vi "LabVIEW_Interface.vi"() -> ()   [LabVIEW 2023]
uses:
  <vilib>/Instr/_visa.llb/VISA Configure Serial Port (Instr).vi
  <vilib>/addons/control/pid/pid.llb/PID (DBL).vi
  <vilib>/addons/control/pid/NI_PID_pid.lvlib
panel:
  in  "PID/Manual control":bool
  in  "Horizontal Pointer time Arduino":i32(slide)=78 scale=20.0..100.0
  out "Microcontroller reading time":dbl(graph)=78.0
  out "Manual control":bool
  out "PID control":bool=TRUE
  in  "Third speed":i32=128 min=0 max=255 step=1
  in  "Second speed":i32=255 min=0 max=255 step=1
  in  "First speed":i32=255 min=0 max=255 step=1
  out "output manual control":i32=255
  out "Status":string="Closing connection."
  in  "PID gains":T1={"Proportional gain (Kp)"=60.0, "Integral time (Ti)"=0.2, "Derivative time (Td)"=0.0} {"Derivative time (Td)" step=0.001; "Integral time (Ti)" step=0.1; "Proportional gain (Kp)" step=0.1}
  out "output PID":i32=26
  out "Last distance value":dbl=7.16
  out "Sent target position value":dbl=7.0
  out "Vertical Graduated Bar":dbl(slide)=7.16 scale=6.0..16.0
  out "Off":bool=TRUE
  in  "Target position":dbl=7.0 min=7.0 max=16.0 step=0.1
  out "Press submit":bool=TRUE
  in  "Submit":bool
  in  "Stop":bool
  out "On":bool
  in  "VISA resource name":refnum<visa-resource-name>="COM3"
  out "Distance from the linear actuator":waveform(dbl)(graph)={"t0"=timestamp(3798521723.060967 s since 1904-01-01), "dt"=1.0, "Y"=[7.16]}
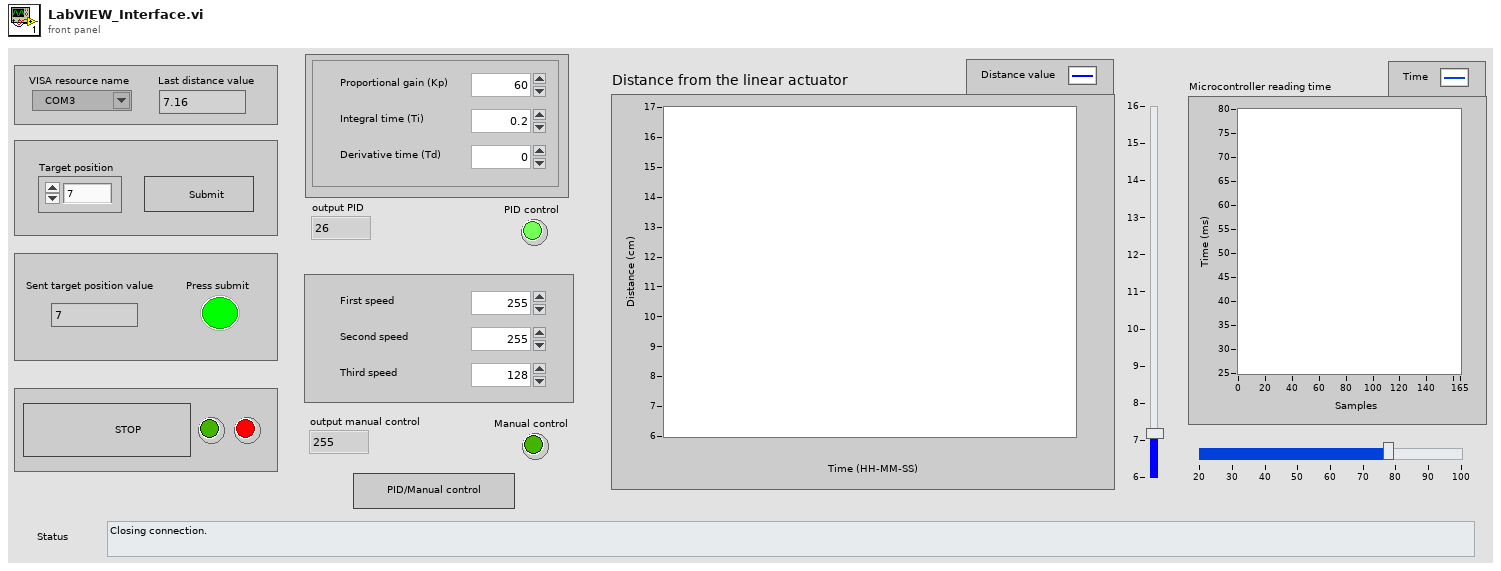
[diagram p1: front panel]
types:
  T1 = cluster{"Proportional gain (Kp)":dbl, "Integral time (Ti)":dbl, "Derivative time (Td)":dbl}
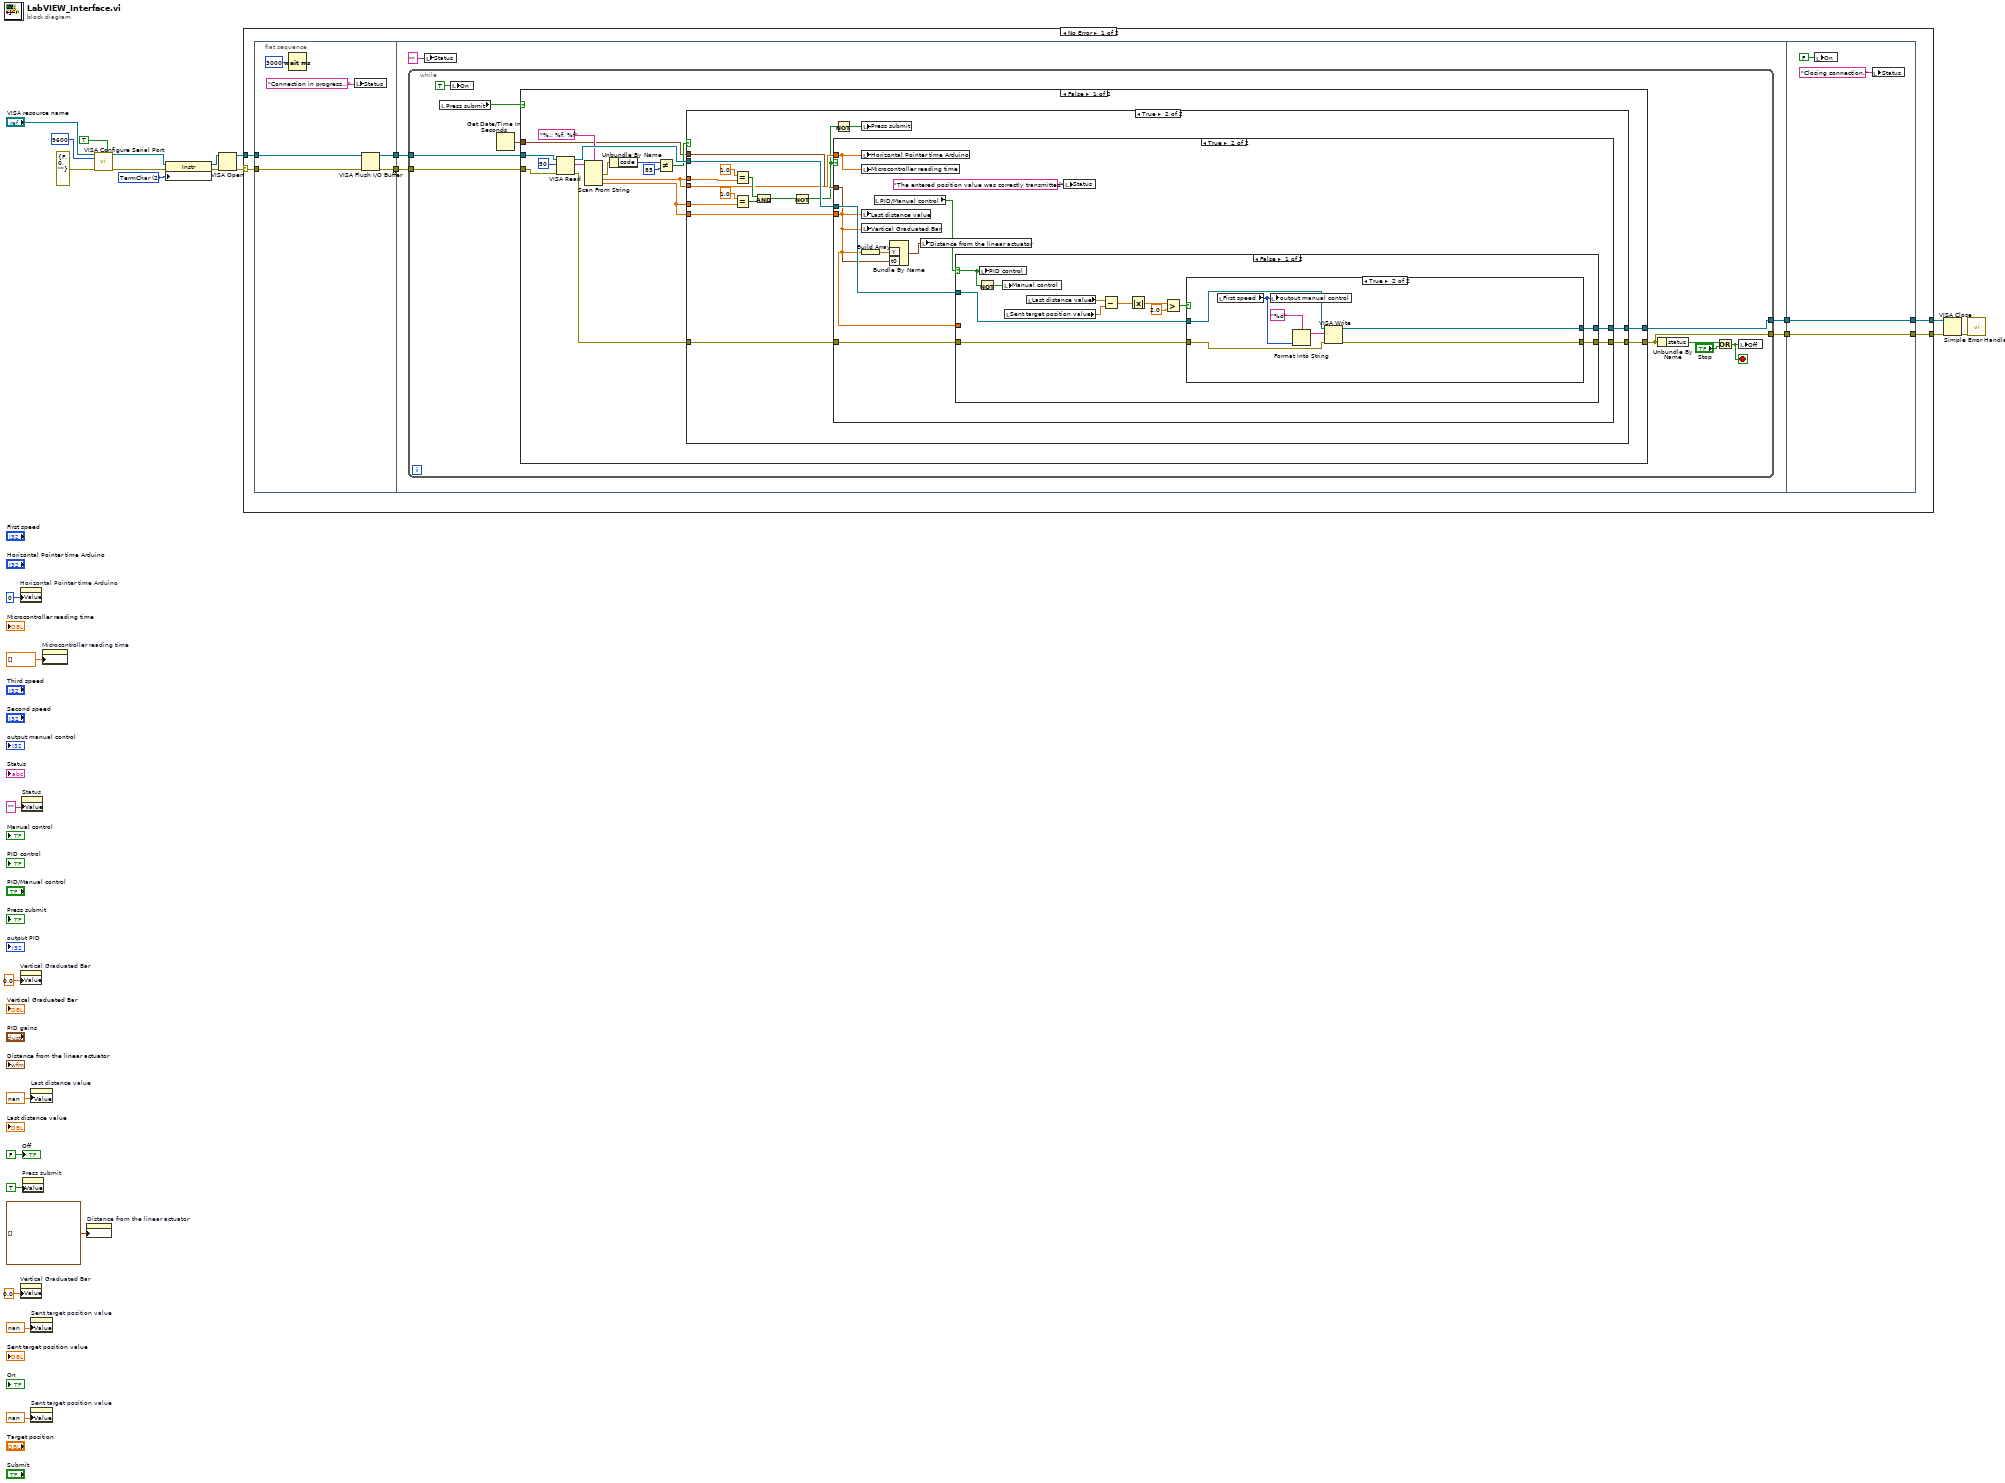
[diagram p0: block diagram]
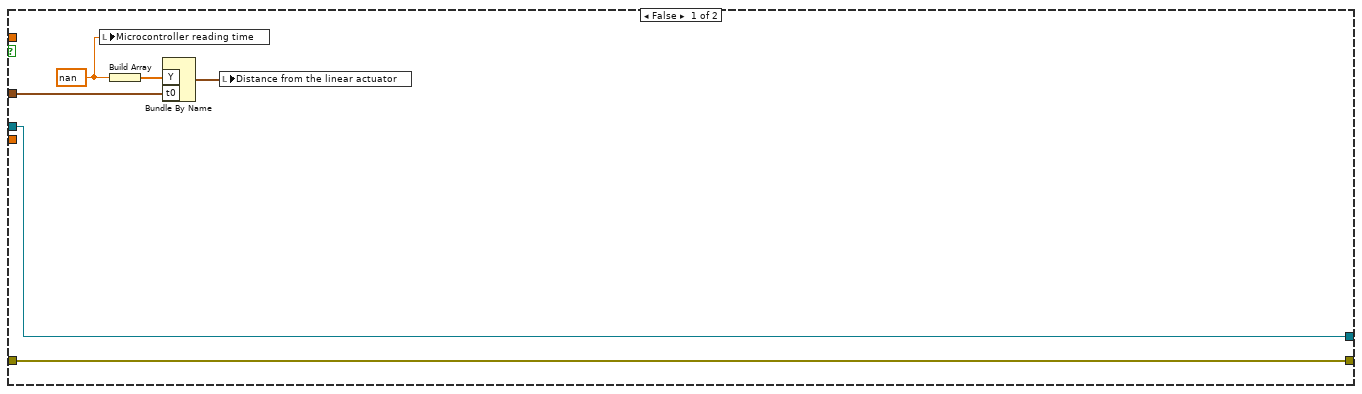
[diagram p3: hidden frame]
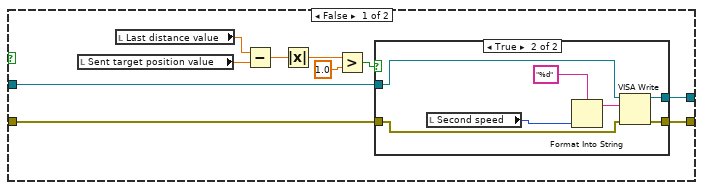
[diagram p4: hidden frame]
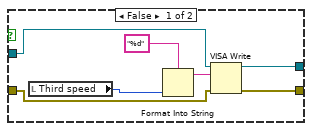
[diagram p5: hidden frame]
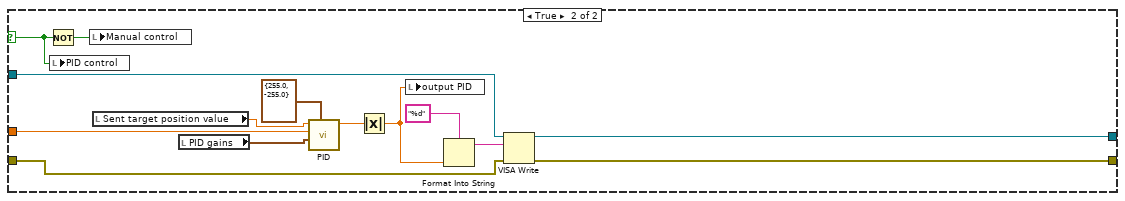
[diagram p6: hidden frame]
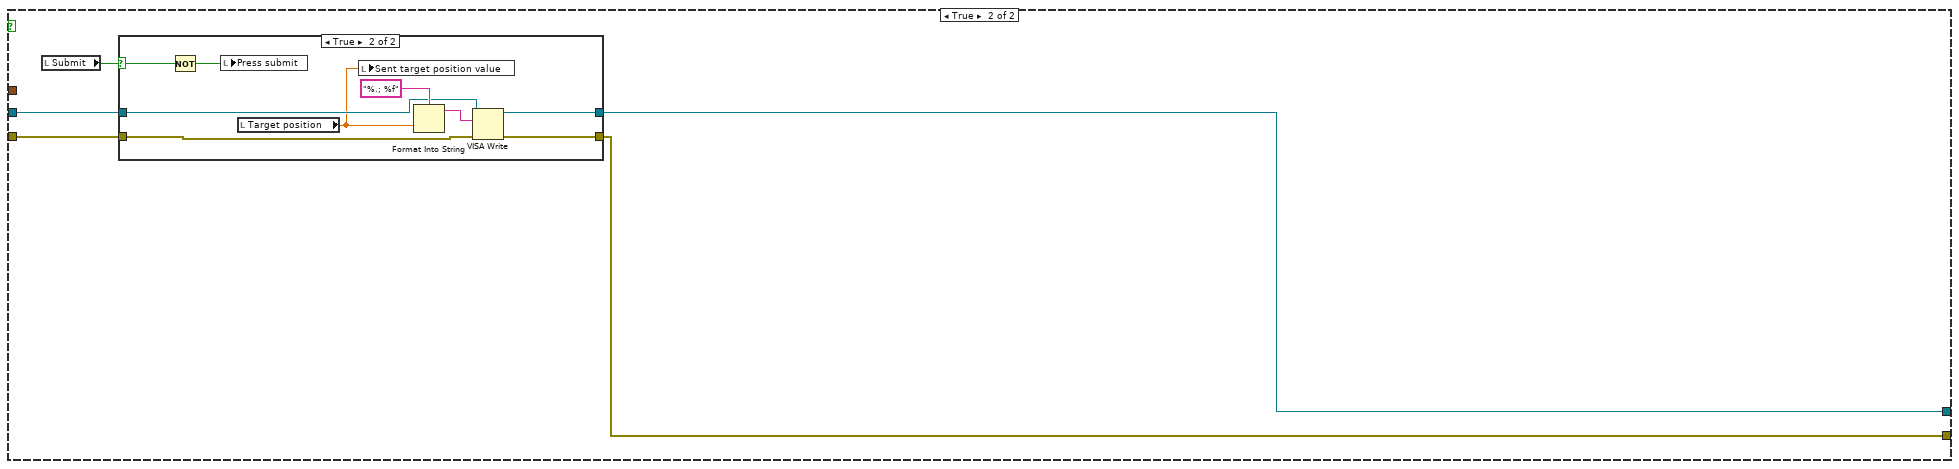
[diagram p7: hidden frame]
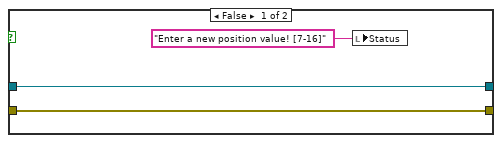
[diagram p8: hidden frame]
diagram:
  w14 = u16 2 items=["None", "LastBit", "TermChar", "Break"] ("Serial Settings:Serial End Mode for Writes")
  n1 = property on="Horizontal Pointer time Arduino" class="Slide (strict)"("Value"=0 ("Horizontal Pointer time Arduino")) -> ()  [unwired: 2 in, 2 out]
  n2 = property on="Vertical Graduated Bar" class="Slide (strict)"("Value"=0.0 ("Vertical Graduated Bar")) -> ()  [unwired: 2 in, 2 out]
  n3 = property on="Vertical Graduated Bar" class="Slide (strict)"("Value"=0.0 ("Vertical Graduated Bar")) -> ()  [unwired: 2 in, 2 out]
  n4 = property on="Status" class="Str"("Value"="" ("Status")) -> ()  [unwired: 2 in, 2 out]
  n5 = property on="Press submit" class="Bool (strict)"("Value"=TRUE ("Press submit")) -> ()  [unwired: 2 in, 2 out]
  n6 = property on="Last distance value" class="DigNum (strict)"("Value"=nan) -> ()  [unwired: 2 in, 2 out]
  n7 = property on="Sent target position value" class="DigNum (strict)"("Value"=nan) -> ()  [unwired: 2 in, 2 out]
  n8 = property on="Sent target position value" class="DigNum (strict)"("Value"=nan) -> ()  [unwired: 2 in, 2 out]
  n9 = property on="Microcontroller reading time" class="WFChart (strict)"("History Data"=dbl[] []) -> ()  [unwired: 2 in, 2 out]
  n10 = property on="Distance from the linear actuator" class="WFChart (strict)"("History Data"=waveform(dbl)[] []) -> ()  [unwired: 2 in, 2 out]
  n11 = call-poly "VISA Configure Serial Port"("VISA resource name"="VISA resource name", "Enable Termination\nChar (T)"=TRUE ("Enable Termination\nChar (T)"), "baud rate (9600)"=u32 9600, "error in (no error)"=errorcluster {"status"=FALSE, "code"=0, "source"=""}) -> ("VISA resource name out"=w13:refnum<visa-resource-name>, "error out"=w12:errorcluster)  [unwired: 10 in]
  n12 = property class="Instr"(reference=w13, error in=w12, "Serial Settings:End Mode for Writes"=w14) -> (reference out=w11:refnum<visa-resource-name>, error out=w10:errorcluster)
  n13 = VISA Open(error in (no error)=w10, VISA resource name=w11) -> (VISA resource name=w21:refnum<visa-resource-name>, error out=w16:errorcluster)  [unwired: 3 in]
  n14 = case shown="No Error" w16 {
    selector: w16 -> [w28 w184]
    tunnel: [w26 w185] -> w23
    tunnel: w21 -> [w30 w185]
    tunnel: [w29 w184] -> w19
    frame No Error {
      n15 = flat-sequence {
        tunnel: w30 -> [w38]
        tunnel: w28 -> [w37]
        tunnel: [w36] -> w33
        tunnel: [w35] -> w32
        tunnel: w33 -> [w44]
        tunnel: w32 -> [w43]
        tunnel: [w42] -> w31
        tunnel: [w41] -> w27
        tunnel: [w183] -> w29
        tunnel: w31 -> [w183]
        tunnel: w27 -> [w181]
        tunnel: [w181] -> w26
        frame #0 {
          n16 = Wait (ms)(milliseconds to wait=u32 3000) -> ()  [unwired: 1 out]
          n17 = local write "Status"("Connection in progress..." ("Status")) -> ()
          n18 = VISA Flush I/O Buffer(VISA resource name=w38, error in (no error)=w37) -> (VISA resource name out=w36:refnum<visa-resource-name>, error out=w35:errorcluster)  [unwired: 1 in]
        }
        frame #1 {
          n19 = while {
            tunnel: w44 -> [w50]
            tunnel: [w49] -> w41
            tunnel: w43 -> [w51]
            tunnel: [w48] -> w42
            stop <- w52 stop-if-true
            n20 = local read "Press submit"() -> (w46:bool)
            n21 = local write "On"(TRUE ("On")) -> ()
            n22 = Get Date/Time In Seconds() -> (seconds since 1Jan1904=w45:timestamp)
            n23 = case shown="False" w46 {
              tunnel: w50 -> [w69 w167]
              tunnel: w51 -> [w68 w166]
              tunnel: [w65 w165] -> w49
              tunnel: [w64 w164] -> w48
              tunnel: w45 -> [w55 _]
              frame False {
                n24 = VISA Read(VISA resource name=w69, byte count=u32 50, error in (no error)=w68) -> (VISA resource name out=w67:refnum<visa-resource-name>, read buffer=w63:string, error out=w66:errorcluster)  [unwired: 1 out]
                n25 = Scan From String(format string="%.; %f, %f", input string=w63) -> (error out=w61:errorcluster, output 1=w56:dbl, output 2=w57:dbl)  [unwired: 4 in, 2 out]
                n26 = Unbundle By Name(w61) -> ("code"=w60:i32)
                n27 = Not Equal?(x=w60, y=85) -> (x != y?=w58:bool)
                n28 = case shown="True" w58 {
                  tunnel: w57 -> [_ w84]
                  tunnel: w67 -> [w71 w88]
                  tunnel: w66 -> [w72 w87]
                  tunnel: [w71 w86] -> w65
                  tunnel: [w72 w85] -> w64
                  tunnel: w56 -> [_ w77]
                  tunnel: w57 -> [_ w76]
                  tunnel: w56 -> [_ w75]
                  tunnel: w55 -> [_ w74]
                  frame False {
                  }
                  frame True {
                    n29 = Equal?(x=1.0, y=w77) -> (x = y?=w81:bool)
                    n30 = Equal?(x=1.0, y=w76) -> (x = y?=w82:bool)
                    n31 = And(x=w81, y=w82) -> (x .and. y?=w83:bool)
                    n32 = Not(x=w83) -> (.not. x?=w73:bool)
                    n33 = case shown="True" w73 {
                      tunnel: w88 -> [w94 w103]
                      tunnel: w87 -> [w93 w102]
                      tunnel: [w94 w101] -> w86
                      tunnel: [w93 w100] -> w85
                      tunnel: w84 -> [_ w97]
                      tunnel: w75 -> [_ w96]
                      tunnel: w74 -> [w91 w95]
                      frame False {
                        w89 = nan
                        n34 = local write "Microcontroller reading time"(w89) -> ()
                        n35 = Build Array(w89) -> (w92:dbl[])
                        n36 = Bundle By Name("Y"=w92, "t0"=w91) -> (w90:waveform(dbl))  [unwired: 1 in]
                        n37 = local write "Distance from the linear actuator"(w90) -> ()
                      }
                      frame True {
                        n38 = local write "Horizontal Pointer time Arduino"(w96) -> ()
                        n39 = local write "Microcontroller reading time"(w96) -> ()
                        n40 = local write "Last distance value"(w97) -> ()
                        n41 = local write "Vertical Graduated Bar"(w97) -> ()
                        n42 = Build Array(w97) -> (w105:dbl[])
                        n43 = local read "PID/Manual control"() -> (w99:bool)
                        n44 = Bundle By Name("Y"=w105, "t0"=w95) -> (w104:waveform(dbl))  [unwired: 1 in]
                        n45 = local write "Distance from the linear actuator"(w104) -> ()
                        n46 = case shown="False" w99 {
                          selector: w99 -> [w113 w151]
                          tunnel: w103 -> [w117 w160]
                          tunnel: w102 -> [w116 w159]
                          tunnel: [w115 w158] -> w101
                          tunnel: [w114 w157] -> w100
                          tunnel: w97 -> [_ w155]
                          frame False {
                            n47 = Not(x=w113) -> (.not. x?=w112:bool)
                            n48 = local write "PID control"(w113) -> ()
                            n49 = local write "Manual control"(w112) -> ()
                            n50 = local read "Sent target position value"() -> (w111:dbl)
                            n51 = local read "Last distance value"() -> (w110:dbl)
                            n52 = Subtract(x=w110, y=w111) -> (x-y=w109:dbl)
                            n53 = Absolute Value(x=w109) -> (abs(x)=w107:dbl)
                            n54 = Greater?(x=w107, y=2.0) -> (0:w106:bool)
                            n55 = case shown="True" w106 {
                              tunnel: w117 -> [w127 w148]
                              tunnel: w116 -> [w126 w147]
                              tunnel: [w125 w146] -> w115
                              tunnel: [w124 w145] -> w114
                              frame False {
                                n56 = local read "Sent target position value"() -> (w121:dbl)
                                n57 = local read "Last distance value"() -> (w122:dbl)
                                n58 = Subtract(x=w122, y=w121) -> (x-y=w120:dbl)
                                n59 = Absolute Value(x=w120) -> (abs(x)=w119:dbl)
                                n60 = Greater?(x=w119, y=1.0) -> (0:w123:bool)
                                n61 = case shown="True" w123 {
                                tunnel: w127 -> [w132 w139]
                                tunnel: w126 -> [w129 w138]
                                tunnel: [w131 w137] -> w125
                                tunnel: [w130 w136] -> w124
                                frame False {
                                n62 = local read "Third speed"() -> (w128:i32)
                                n63 = Format Into String(format string="%d", w128) -> (resulting string=w133:string)  [unwired: 2 in, 1 out]
                                n64 = VISA Write(VISA resource name=w132, write buffer=w133, error in (no error)=w129) -> (VISA resource name out=w131:refnum<visa-resource-name>, error out=w130:errorcluster)  [unwired: 1 out]
                                }
                                frame True {
                                n65 = local read "Second speed"() -> (w135:i32)
                                n66 = Format Into String(format string="%d", w135) -> (resulting string=w140:string)  [unwired: 2 in, 1 out]
                                n67 = VISA Write(VISA resource name=w139, write buffer=w140, error in (no error)=w138) -> (VISA resource name out=w137:refnum<visa-resource-name>, error out=w136:errorcluster)  [unwired: 1 out]
                                }
                                }
                              }
                              frame True {
                                n68 = local read "First speed"() -> (w142:i32)
                                n69 = local write "output manual control"(w142) -> ()
                                n70 = Format Into String(format string="%d", w142) -> (resulting string=w144:string)  [unwired: 2 in, 1 out]
                                n71 = VISA Write(VISA resource name=w148, write buffer=w144, error in (no error)=w147) -> (VISA resource name out=w146:refnum<visa-resource-name>, error out=w145:errorcluster)  [unwired: 1 out]
                              }
                            }
                          }
                          frame True {
                            n72 = Not(x=w151) -> (.not. x?=w152:bool)
                            n73 = local write "PID control"(w151) -> ()
                            n74 = local write "Manual control"(w152) -> ()
                            n75 = local read "Sent target position value"() -> (w154:dbl)
                            n76 = local read "PID gains"() -> (w153:T1)
                            n77 = call-poly <vilib>:"PID.vi"("output range"=cluster{"output high":dbl, "output low":dbl} {"output high"=255.0, "output low"=-255.0}, "PID gains"=w153, "process variable"=w155, "setpoint"=w154) -> ("output"=w150:dbl)  [unwired: 6 in, 1 out]
                            n78 = Absolute Value(x=w150) -> (abs(x)=w149:dbl)
                            n79 = local write "output PID"(w149) -> ()
                            n80 = Format Into String(format string="%d", w149) -> (resulting string=w161:string)  [unwired: 2 in, 1 out]
                            n81 = VISA Write(VISA resource name=w160, write buffer=w161, error in (no error)=w159) -> (VISA resource name out=w158:refnum<visa-resource-name>, error out=w157:errorcluster)  [unwired: 1 out]
                          }
                        }
                        n82 = local write "Status"("The entered position value was correctly transmitted" ("String 2")) -> ()
                      }
                    }
                    n83 = Not(x=w73) -> (.not. x?=w78:bool)
                    n84 = local write "Press submit"(w78) -> ()
                  }
                }
              }
              frame True {
                n85 = local read "Submit"() -> (w163:bool)
                n86 = case shown="True" w163 {
                  selector: w163 -> [_ w172]
                  tunnel: w167 -> [w170 w178]
                  tunnel: w166 -> [w169 w177]
                  tunnel: [w170 w174] -> w165
                  tunnel: [w169 w173] -> w164
                  frame False {
                    n87 = local write "Status"("Enter a new position value! [7-16]" ("Status")) -> ()
                  }
                  frame True {
                    n88 = Not(x=w172) -> (.not. x?=w171:bool)
                    n89 = local write "Press submit"(w171) -> ()
                    n90 = local read "Target position"() -> (w175:dbl)
                    n91 = local write "Sent target position value"(w175) -> ()
                    n92 = Format Into String(format string="%.; %f", w175) -> (resulting string=w176:string)  [unwired: 2 in, 1 out]
                    n93 = VISA Write(VISA resource name=w178, write buffer=w176, error in (no error)=w177) -> (VISA resource name out=w174:refnum<visa-resource-name>, error out=w173:errorcluster)  [unwired: 1 out]
                  }
                }
              }
            }
            n94 = Unbundle By Name(w48) -> ("status"=w54:bool)
            n95 = Or(x=w54, y="Stop") -> (x .or. y?=w52:bool)
            n96 = local write "Off"(w52) -> ()
          }
          n97 = local write "Status"("" ("Status")) -> ()
        }
        frame #2 {
          n98 = local write "On"(FALSE ("On")) -> ()
          n99 = local write "Status"("Closing connection." ("Status")) -> ()
        }
      }
    }
    frame Error {
    }
  }
  n100 = VISA Close(VISA resource name=w23, error in (no error)=w19) -> (error out=w18:errorcluster)
  n101 = call <vilib>:"Simple Error Handler.vi"("error in (no error)"=w18) -> ()  [unwired: 4 in, 5 out]
  "Off" <- FALSE ("Off")
